vi "Begin.vi"() -> (0 "error out 2":errorcluster, 1 "Co_fifo":refnum<k33>, 2 "drive log":refnum<file>, 3 "Drive_fifo":refnum<k33>)   [LabVIEW 2014]
doc: "Called before other user functions, this VI is expected to open initial I/O refnums, load in file data, and do all program initialization. Notice that the <B>error out</B> terminal is simply used for data flow. Wiring it to other structures or subVIs ensures that this VI runs first."
uses:
  Lightning base/TeleopCmd.ctl
  Lightning base/CmdFlag.ctl
  Lightning base/Co-Pilot_game_control.ctl
  <vilib>/Rock Robotics/WPI/DriverStation/WPI_DriverStationRobotMode2.ctl
  Robot Global Data.vi
panel:
  in  "error in (no error)":errorcluster
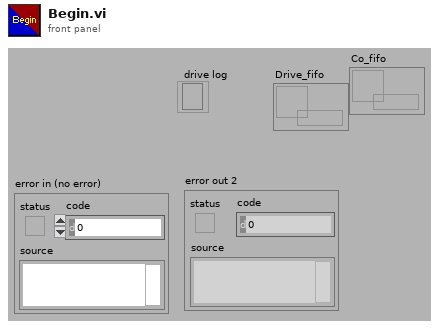
[diagram p1: front panel]
types:
  T1 = typedef "Co-Pilot_game_control.ctl" = cluster{"Left_Intake":dbl, "Right_Intake":dbl, "Time Stamp":dbl}
  T2 = enum16{"open", "replace", "create", "open or create", "replace or create", "replace or create with confirmation"}
  T3 = typedef "TeleopCmd.ctl" = cluster{"CmdFlag":T4, "throttle":dbl, "turn":dbl, "Override":bool, "Strafe":dbl, "MotorPwrMax":u8, "Time":u32}
  T4 = typedef "CmdFlag.ctl" = enum16{"noop", "suspend", "resume"}
  T5 = typedef "WPI_DriverStationRobotMode2.ctl" = enum16{"Autonomous Disabled", "Autonomous Enabled", "Teleop Disabled", "Teleop Enabled", "Disconnected", "Finish", "Test Disabled", "Test Enabled", "Emergency Stopped"}
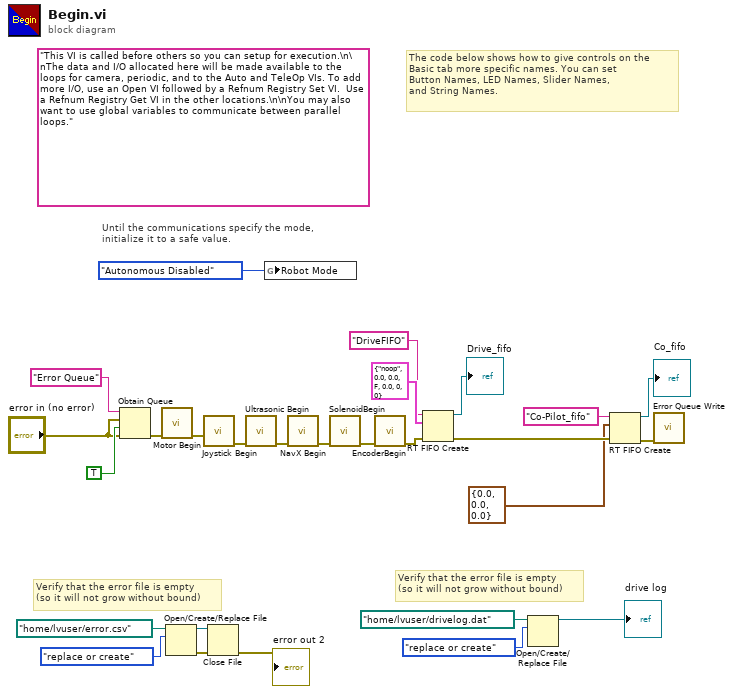
[diagram p0: block diagram]
diagram:
  (unwired) "This VI is called before others so you can setup for execution.\n\nThe data and I/O allocated here will be made available to the loops for camera, periodic, and to the Auto and TeleOp VIs. To add more I/O, use an Open VI followed by a Refnum Registry Set VI.  Use a Refnum Registry Get VI in the other locations.\n\nYou may also want to use global variables to communicate between parallel loops."
  # "Verify that the error file is empty \n(so it will not grow without bound)"
  # "Verify that the error file is empty \n(so it will not grow without bound)"
  # "The code below shows how to give controls on the\nBasic tab more specific names. You can set\nButton Names, LED Names, Slider Names,\nand String Names."
  # "Until the communications specify the mode,\ninitialize it to a safe value."
  n1 = Obtain Queue(name (unnamed)="Error Queue", element data type="error in (no error)", create if not found? (T)=TRUE, error in (no error)="error in (no error)") -> (error out=w13:errorcluster)  [unwired: 1 in, 2 out]
  n2 = call "Motor Begin.vi"("error in (no error)"=w13) -> ("error out"=w26:errorcluster)  [unwired: 10 in]
  n3 = Open/Create/Replace File(file path (use dialog)=path "/home/lvuser/error.csv", operation (0:open)=T2."replace or create") -> (refnum out=w18:refnum<file>, error out=w17:errorcluster)  [unwired: 4 in, 1 out]
  n4 = call "Joystick Begin.vi"("error in (no error)"=w26) -> ("error out"=w8:errorcluster)  [unwired: 10 in]
  n5 = Close File(refnum=w18, error in=w17) -> (error out=→"error out 2":errorcluster)  [unwired: 1 out]
  n6 = call "Ultrasonic Begin.vi"("error in"=w8) -> ("error out"=w7:errorcluster)  [unwired: 10 in]
  n7 = global write "Robot Global Data.vi" "Robot Mode"(WPI_DriverStationRobotMode2."Autonomous Disabled" ("Robot Mode")) -> ()
  n8 = call "NavX Begin.vi"("error in"=w7) -> ("error out"=w6:errorcluster)  [unwired: 10 in]
  n9 = call "SolenoidBegin.vi"("error in (no error)"=w6) -> ("error out"=w25:errorcluster)  [unwired: 10 in]
  n10 = call "EncoderBegin.vi"("error in (no error)"=w25) -> ("error out"=w22:errorcluster)  [unwired: 10 in]
  n11 = RT FIFO Create(0:"DriveFIFO" ("name (unnamed)"), 1:T3 {"CmdFlag"=enum."noop", "throttle"=0.0, "turn"=0.0, "Override"=FALSE, "Strafe"=0.0, "MotorPwrMax"=0, "Time"=0} ("Cluster"), 3:w22) -> (8:→"Drive_fifo":refnum<k33>, 11:w5:errorcluster)  [unwired: 5 in, 1 out]
  n12 = Open/Create/Replace File(file path (use dialog)=path "/home/lvuser/drivelog.dat", operation (0:open)=T2."replace or create") -> (refnum out=→"drive log":refnum<file>)  [unwired: 4 in, 2 out]
  n13 = RT FIFO Create(0:"Co-Pilot_fifo" ("name (unnamed)"), 1:T1 {"Left_Intake"=0.0, "Right_Intake"=0.0, "Time Stamp"=0.0}, 3:w5) -> (8:→"Co_fifo":refnum<k33>, 11:w4:errorcluster)  [unwired: 5 in, 1 out]
  n14 = call "Error Queue Write.vi"("error in (no error)"=w4) -> ()  [unwired: 11 in]
